vi "Day01-05.vi"() -> ()   [LabVIEW 2021]
panel:
  out "x-y":u32
  out "ms 타이머 값":u32
  in  "정지 5":bool
  in  "정지 4":bool
  in  "정지 3":bool
  out "숫자형 3":i32
  out "숫자형 2":i32
  out "숫자형":i32
  out "x+y 2":dbl
  in  "정지 2":bool
  out "x+y":dbl
  in  "정지":bool
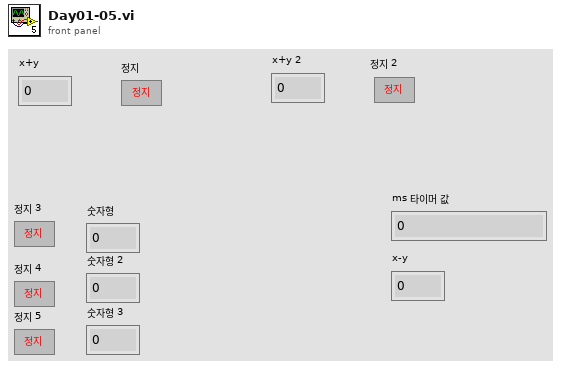
[diagram p1: front panel]
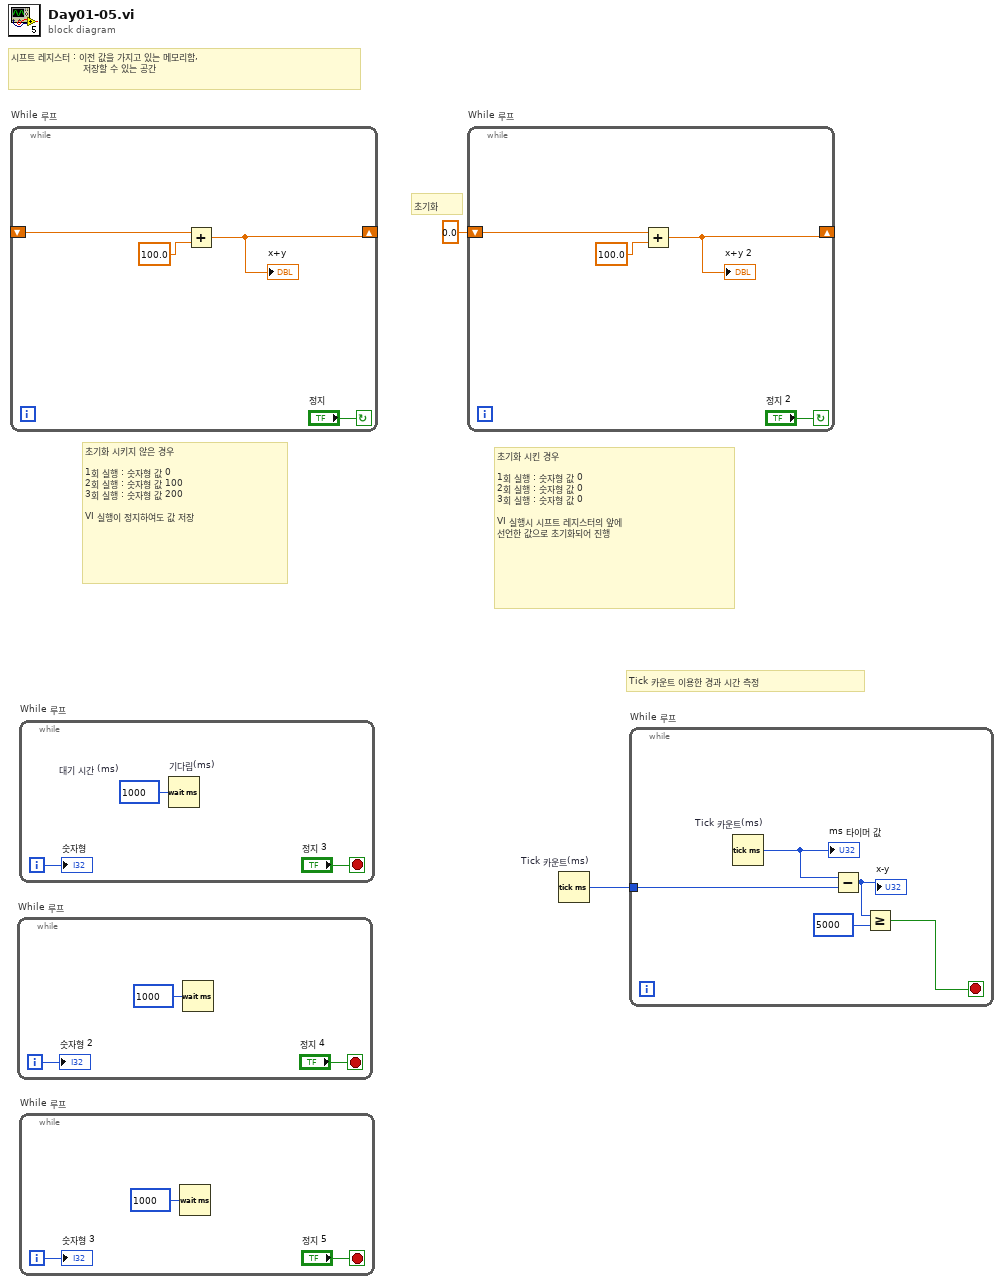
[diagram p0: block diagram]
diagram:
  # "Tick 카운트 이용한 경과 시간 측정"
  # "초기화 시킨 경우\n\n1회 실행 : 숫자형 값 0\n2회 실행 : 숫자형 값 0\n3회 실행 : 숫자형 값 0\n\nVI 실행시 시프트 레지스터의 앞에 \n선언한 값으로 초기화되어 진행"
  # "초기화 시키지 않은 경우\n\n1회 실행 : 숫자형 값 0\n2회 실행 : 숫자형 값 100\n3회 실행 : 숫자형 값 200\n\nVI 실행이 정지하여도 값 저장"
  # "초기화"
  # "시프트 레지스터 : 이전 값을 가지고 있는 메모리함, \n                        저장할 수 있는 공간"
  n1 = while "While 루프" {
    shift-right: [w4] -> _
    shift-left: _ -> [w6]
    stop <- "정지" continue-if-true
    n2 = Add(x=w6, y=100.0) -> (x+y=w4:dbl)
    "x+y" <- w4
  }
  n3 = while "While 루프" {
    i -> [w9]
    stop <- "정지 4" stop-if-true
    n4 = Wait (ms) ("기다림(ms)")(milliseconds to wait=u32 1000 ("대기 시간 (ms)")) -> ()  [unwired: 1 out]
    "숫자형 2" <- w9
  }
  n5 = while "While 루프" {
    i -> [w12]
    stop <- "정지 3" stop-if-true
    w10 = u32 1000  # 대기 시간 (ms)
    n6 = Wait (ms) "기다림(ms)"(milliseconds to wait=w10) -> ()  [unwired: 1 out]
    "숫자형" <- w12
  }
  n7 = while "While 루프" {
    i -> [w15]
    stop <- "정지 5" stop-if-true
    n8 = Wait (ms) ("기다림(ms)")(milliseconds to wait=u32 1000 ("대기 시간 (ms)")) -> ()  [unwired: 1 out]
    "숫자형 3" <- w15
  }
  n9 = while "While 루프" {
    shift-right: [w17] -> _
    shift-left: 0.0 -> [w19]
    stop <- "정지 2" continue-if-true
    n10 = Add(x=w19, y=100.0) -> (x+y=w17:dbl)
    "x+y 2" <- w17
  }
  n11 = Tick Count (ms) "Tick 카운트(ms)"() -> (millisecond timer value=w1:u32)
  n12 = while "While 루프" {
    tunnel: w1 -> [w24]
    stop <- w20 stop-if-true
    n13 = Tick Count (ms) "Tick 카운트(ms)"() -> (millisecond timer value=w23:u32)
    "ms 타이머 값" <- w23
    n14 = Subtract(x=w23, y=w24) -> (x-y=w22:u32)
    "x-y" <- w22
    n15 = Greater Or Equal?(x=w22, y=u32 5000) -> (x >= y?=w20:bool)
  }
